vi "rd_initialTimeStampFormat.vi"(8 "error in (no error)":errorcluster, 11 "timestamp format":string) -> (0 "error out":errorcluster, 3 "timestamp format out":string)   [LabVIEW 2017, in "NI_ExcelFile.lvlib"]
uses:
  <vilib>/express/express shared/NI_ExcelFile/NI_ExcelFile.lvlib
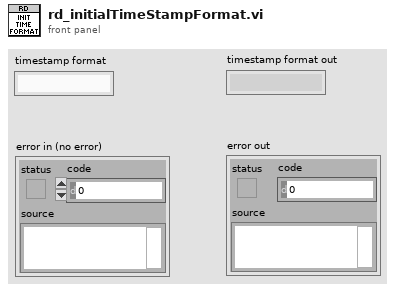
[diagram p1: front panel]
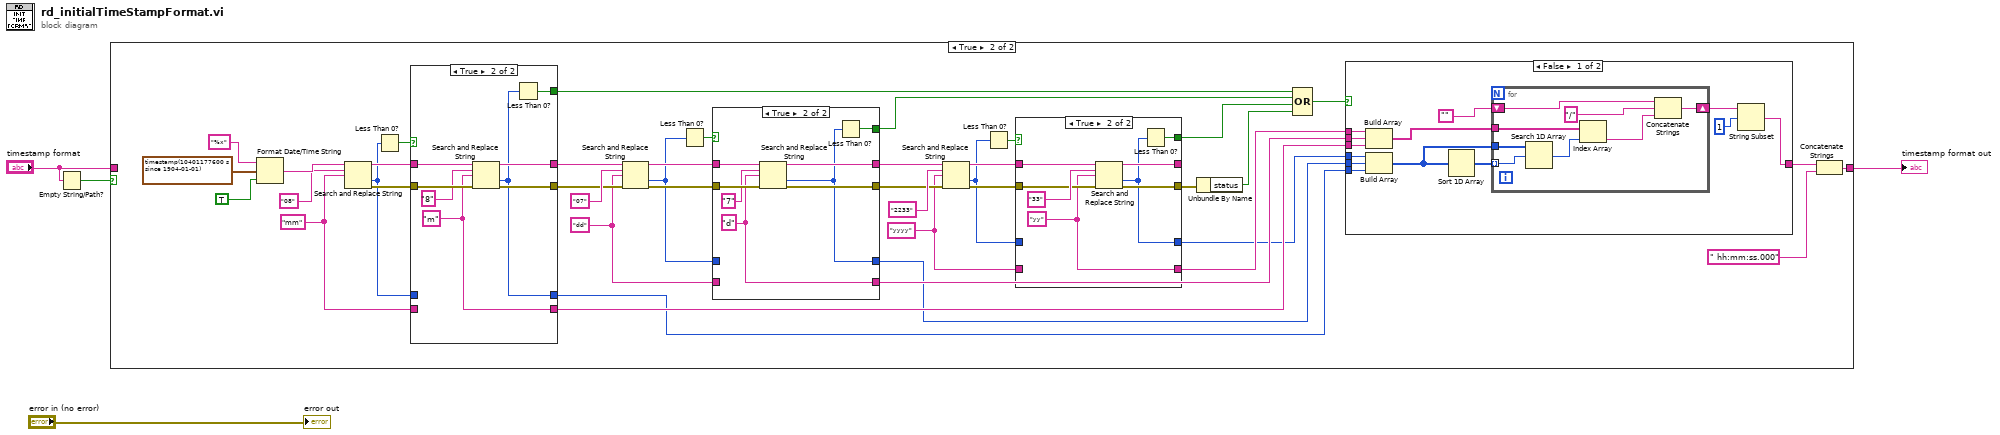
[diagram p0: block diagram]
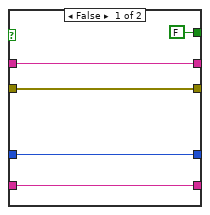
[diagram p3: hidden frame]
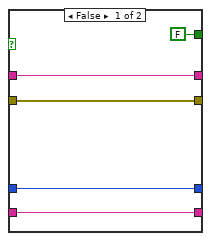
[diagram p4: hidden frame]
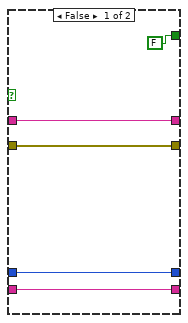
[diagram p5: hidden frame]
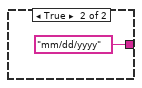
[diagram p6: hidden frame]
diagram:
  n1 = Empty String/Path?(string/path="timestamp format") -> (empty?=w4:bool)
  n2 = case shown="True" w4 {
    tunnel: [w5 w21] -> w2
    tunnel: "timestamp format" -> [w5 _]
    frame False {
    }
    frame True {
      w12 = "yyyy" ("replace string (\"\")")
      w15 = "dd" ("replace string (\"\")")
      w19 = "mm" ("replace string (\"\")")
      n3 = Format Date/Time String(time format string (%c)="%x" ("format string"), seconds (now)=timestamp(10401177600.001 s since 1904-01-01), UTC format=TRUE) -> (date/time string=w45:string)
      n4 = Search and Replace String(input string=w45, search string="08", replace string=w19) -> (result string=w38:string, offset past replacement=w18:i32, error out=w37:errorcluster)  [unwired: 5 in, 1 out]
      n5 = Less Than 0?(x=w18) -> (x < 0?=w39:bool)
      n6 = case shown="True" w39 {
        tunnel: w38 -> [w77 w85]
        tunnel: w37 -> [w76 w84]
        tunnel: [w76 w82] -> w36
        tunnel: [w77 w81] -> w35
        tunnel: [FALSE w80] -> w34
        tunnel: [w73 w79] -> w6
        tunnel: w19 -> [w74 _]
        tunnel: [w74 w78] -> w9
        tunnel: w18 -> [w73 _]
        frame False {
        }
        frame True {
          w78 = "m" ("replace string (\"\")")
          n7 = Search and Replace String(input string=w85, search string="8", replace string=w78, error in=w84) -> (result string=w81:string, offset past replacement=w79:i32, error out=w82:errorcluster)  [unwired: 4 in, 1 out]
          n8 = Less Than 0?(x=w79) -> (x < 0?=w80:bool)
        }
      }
      n9 = Search and Replace String(input string=w35, search string="07", replace string=w15, error in=w36) -> (result string=w32:string, offset past replacement=w14:i32, error out=w31:errorcluster)  [unwired: 4 in, 1 out]
      n10 = Less Than 0?(x=w14) -> (x < 0?=w33:bool)
      n11 = case shown="True" w33 {
        tunnel: w32 -> [w64 w72]
        tunnel: w31 -> [w63 w71]
        tunnel: [w63 w69] -> w30
        tunnel: [w64 w68] -> w29
        tunnel: [FALSE w67] -> w28
        tunnel: [w60 w66] -> w7
        tunnel: [w61 w65] -> w10
        tunnel: w15 -> [w61 _]
        tunnel: w14 -> [w60 _]
        frame False {
        }
        frame True {
          w65 = "d" ("replace string (\"\")")
          n12 = Search and Replace String(input string=w72, search string="7", replace string=w65, error in=w71) -> (result string=w68:string, offset past replacement=w66:i32, error out=w69:errorcluster)  [unwired: 4 in, 1 out]
          n13 = Less Than 0?(x=w66) -> (x < 0?=w67:bool)
        }
      }
      n14 = Search and Replace String(input string=w29, search string="2233", replace string=w12, error in=w30) -> (result string=w41:string, offset past replacement=w13:i32, error out=w27:errorcluster)  [unwired: 4 in, 1 out]
      n15 = Less Than 0?(x=w13) -> (x < 0?=w26:bool)
      n16 = case shown="True" w26 {
        tunnel: w41 -> [w50 w59]
        tunnel: w27 -> [w49 w57]
        tunnel: [FALSE w56] -> w25
        tunnel: [w50 w55] -> _
        tunnel: [w49 w54] -> w24
        tunnel: [w48 w53] -> w8
        tunnel: [w47 w52] -> w11
        tunnel: w13 -> [w48 _]
        tunnel: w12 -> [w47 _]
        frame False {
        }
        frame True {
          w52 = "yy" ("replace string (\"\")")
          n17 = Search and Replace String(input string=w59, search string="33", replace string=w52, error in=w57) -> (result string=w55:string, offset past replacement=w53:i32, error out=w54:errorcluster)  [unwired: 4 in, 1 out]
          n18 = Less Than 0?(x=w53) -> (x < 0?=w56:bool)
        }
      }
      n19 = Unbundle By Name(w24) -> ("status"=w23:bool)
      n20 = Compound Arithmetic op=OR(w34, w28, w25, w23) -> (w40:bool)
      n21 = case shown="False" w40 {
        tunnel: [w86 "mm/dd/yyyy" ("timeStamp format")] -> w22
        tunnel: w11 -> [w92 _]
        tunnel: w10 -> [w91 _]
        tunnel: w9 -> [w90 _]
        tunnel: w8 -> [w89 _]
        tunnel: w7 -> [w88 _]
        tunnel: w6 -> [w87 _]
        frame False {
          n22 = Build Array(w92, w91, w90) -> (w94:string[])
          n23 = Build Array(w89, w88, w87) -> (w95:i32[])
          n24 = Sort 1D Array(array=w95) -> (sorted array=w93:i32[])
          n25 = for {
            tunnel: w93 -> [w105] mode=indexing
            tunnel: w94 -> [w104]
            tunnel: w95 -> [w106]
            shift-right: [w101] -> w97
            shift-left: "" -> [w102]
            n26 = Search 1D Array(1D array=w106, element=w105) -> (index of element=w103:i32)  [unwired: 1 in]
            n27 = Index Array(array=w104, index=w103) -> (element=w99:string)
            n28 = Concatenate Strings(w102, "/" ("string"), w99) -> (w101:string)
          }
          n29 = String Subset(string=w97, offset (0)=1) -> (substring=w86:string)  [unwired: 1 in]
        }
        frame True {
        }
      }
      n30 = Concatenate Strings(w22, " hh:mm:ss.000") -> (w21:string)
    }
  }
  "timestamp format out" <- w2
  "error out" <- "error in (no error)"
